vi "Test for Speaker PWM.vi"() -> ()   [LabVIEW 2025]
uses:
  <vilib>/rvi/DesktopExecutionNode/DesktopExecutionNode.xnode
  <vilib>/rvi/DesktopExecutionNode/Execution/niFpgaDEN_Execute.vi
panel:
  in  "Duty Cycle On":u16
  in  "Duty Cycle Off":u16
  out "Mod1/DO0":bool
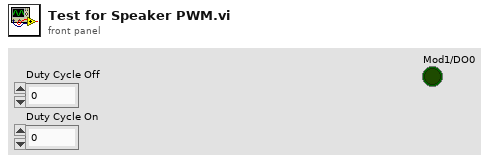
[diagram p1: front panel]
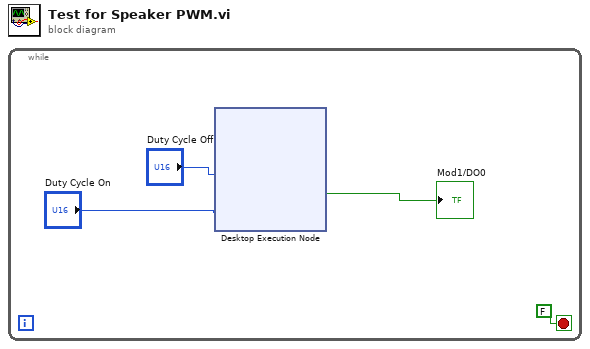
[diagram p0: block diagram]
diagram:
  n1 = while {
    stop <- FALSE ("stop") stop-if-true
    n2 = xnode "Desktop Execution Node"("Duty Cycle On"="Duty Cycle Off", "Duty Cycle Off"="Duty Cycle On") -> ("Mod1/DO0"=→"Mod1/DO0":bool)  [unwired: 1 in, 1 out]
  }
